vi "Gen_ISH_data.vi"(5 "Исходные данные":T1) -> (2 "Исходные tbl":string[][](table))   [LabVIEW 2018]
panel:
  # "Образец"
  # "Параметры КС"
  # "Параметры эксперимента"
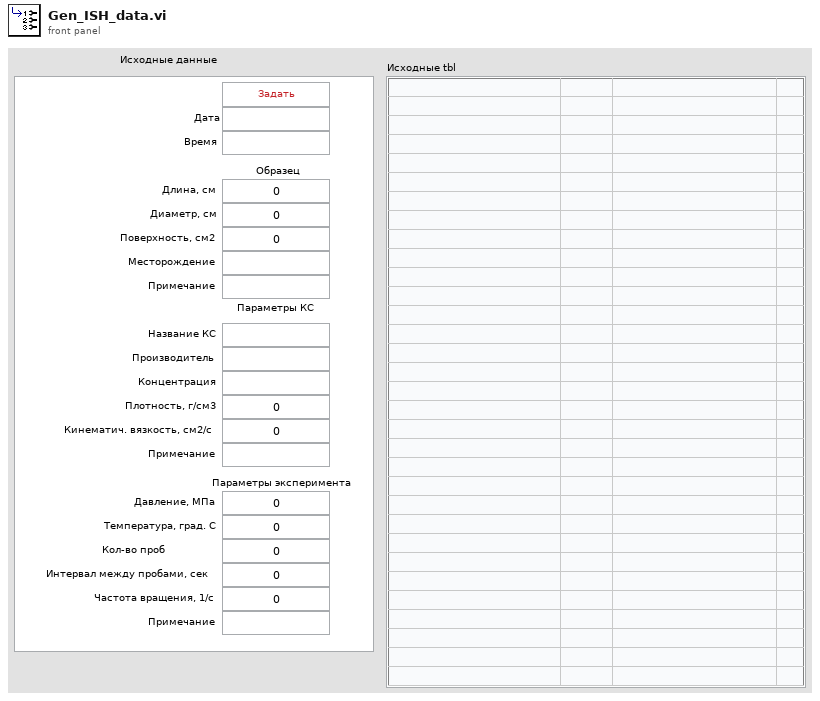
[diagram p1: front panel]
types:
  T1 = typedef "Исходные данные.ctl" = cluster{"Дата":string, "Время":string, "Длина, см ":dbl, "Диаметр, см":dbl, "Поверхность, см2":dbl, "Месторождение":string, "Примечание":string, "Название КС":string, "Производитель":string, "Концентрация":string, "Плотность, г/см3":dbl, "Кинематич. вязкость, см2/с":dbl, "Примечание":string, "Давление, МПа":dbl, "Температура, град. С":dbl, "Кол-во проб":dbl, "Интервал между пробами, сек":dbl, "Частота вращения, 1/с":dbl, "Примечание":string, "Set data":bool}
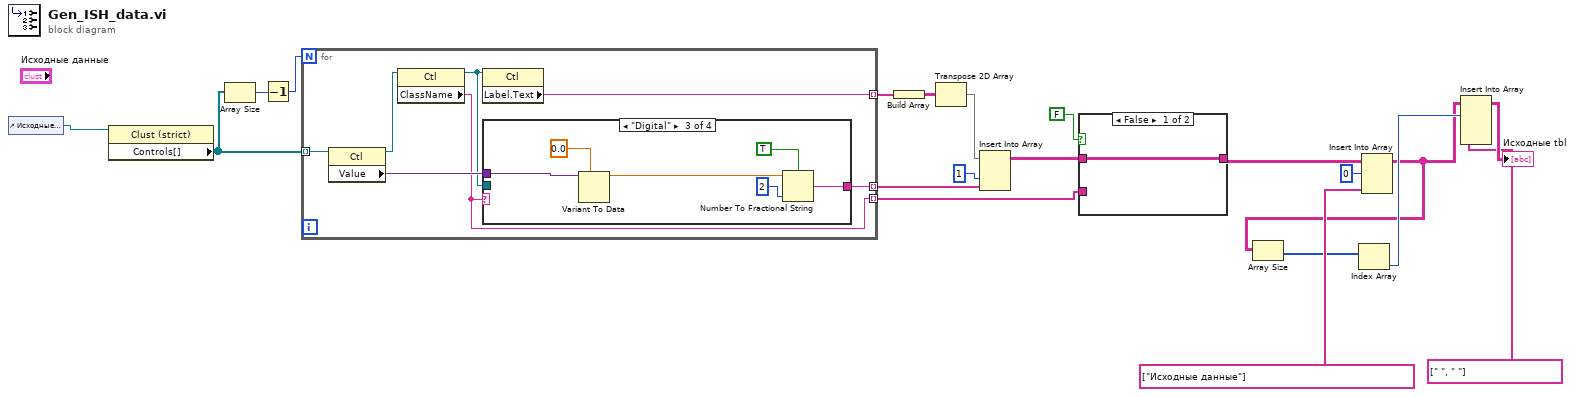
[diagram p0: block diagram]
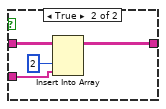
[diagram p2: hidden frame]
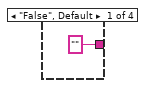
[diagram p3: hidden frame]
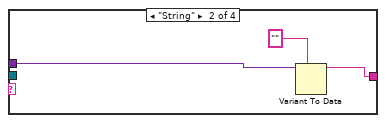
[diagram p4: hidden frame]
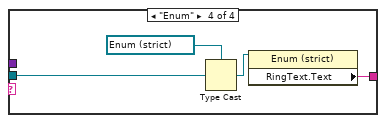
[diagram p5: hidden frame]
diagram:
  w5 = string[] [" ", " "] ("new element/subarray")
  n1 = control-ref of="Исходные данные"() -> (w4:refnum<vi>)
  n2 = property class="Clust (strict)"(reference=w4) -> ("Controls[]"=w3:refnum<vi>[])  [unwired: 1 in, 2 out]
  n3 = Array Size(array=w3) -> (size(s)=w2:i32)
  n4 = Decrement(x=w2) -> (x-1=w1:i32)
  n5 = for {
    N: w1 -> [_]
    tunnel: [w24] -> w19 mode=indexing
    tunnel: w3 -> [w25] mode=indexing
    tunnel: [w23] -> w18 mode=indexing
    tunnel: [w22] -> w14 mode=indexing
    n6 = property class="Ctl"(reference=w25) -> (reference out=w26:refnum<vi>, "Value"=w27:variant)  [unwired: 1 in, 1 out]
    n7 = property class="Ctl"(reference=w26) -> (reference out=w21:refnum<vi>, "ClassName"=w22:string)  [unwired: 1 in, 1 out]
    n8 = property class="Ctl"(reference=w21) -> ("Label.Text"=w23:string)  [unwired: 1 in, 2 out]
    n9 = case shown="\"Digital\"" w22 {
      tunnel: w27 -> [_ w30 w37 _]
      tunnel: ["" w29 w34 w39] -> w24
      tunnel: w21 -> [_ _ _ w41]
      frame "False", Default {
      }
      frame "String" {
        n10 = Variant To Data(type="", Variant=w30) -> (data=w29:string)  [unwired: 1 in, 1 out]
      }
      frame "Digital" {
        n11 = Variant To Data(type=0.0, Variant=w37) -> (data=w35:dbl)  [unwired: 1 in, 1 out]
        n12 = Number To Fractional String(use system decimal point (T)=TRUE, number=w35, precision (6)=i16 2) -> (F-format string=w34:string)  [unwired: 1 in]
      }
      frame "Enum" {
        n13 = Type Cast(type=refnum<vi> refnum ("Enum"), x=w41) -> (*(type *) &x=w40:refnum<vi>)
        n14 = property class="Enum (strict)"(reference=w40) -> ("RingText.Text"=w39:string)  [unwired: 1 in, 2 out]
      }
    }
  }
  n15 = Build Array(w18) -> (w17:string[][])
  n16 = Transpose 2D Array(2D array=w17) -> (transposed array=w16:string[][])
  n17 = Insert Into Array "Insert Into Array"(array=w16, index (col)=1 ("disabled index (col)"), new element=w19) -> (w15:string[][])  [unwired: 1 in]
  n18 = case shown="False" FALSE {
    tunnel: w15 -> [w42 w46]
    tunnel: w14 -> [_ w44]
    tunnel: [w42 w43] -> w10
    frame False {
    }
    frame True {
      n19 = Insert Into Array "Insert Into Array"(array=w46, index (col)=2 ("disabled index (col)"), new element=w44) -> (w43:string[][])  [unwired: 1 in]
    }
  }
  n20 = Insert Into Array "Insert Into Array"(array=w10, index (row)=0, new element=string[] ["Исходные данные"] ("new element/subarray")) -> (w6:string[][])  [unwired: 1 in]
  n21 = Array Size(array=w6) -> (size(s)=w8:i32[])
  n22 = Index Array(array=w8) -> (element=w7:i32)  [unwired: 1 in]
  n23 = Insert Into Array "Insert Into Array"(array=w6, index (row)=w7, new element #1=w5, new element #2=w5) -> (→"Исходные tbl":string[][])  [unwired: 1 in]
